vi "MCLB_AssertAllItems_Tests.vi"(11 "error in":errorcluster) -> (15 "error out":errorcluster)   [LabVIEW 2016, in "DronaTest.lvlib"]
uses:
  DronaTest.lvlib
  APIs/Stimulus/ControlValue/SetValueAuto.vi
  APIs/Assert/AssertControlValue/Controls/MC Listbox/AssertAllItems.vi
  <vilib>/addons/_JKI Toolkits/Caraya/classes/Assert/Assert Error.vi
  <vilib>/addons/_JKI Toolkits/Caraya/classes/Assert/Assert Equal Value_Variant.vi
  <vilib>/addons/_JKI Toolkits/Caraya/classes/Test/Test.lvclass
  Drona.lvlib
  <vilib>/SLL Toolkit/SLL Debug/SLL Debug.lvlib
  <vilib>/addons/_JKI Toolkits/Caraya/classes/Assert/Assert.lvclass
  APIs/Stimulus/ControlValue/ControlValue.lvlib
  APIs/Assert/AssertControlValue/Controls/MC Listbox/AssertMCListbox.lvlib
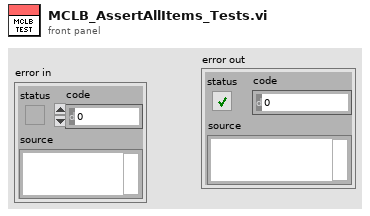
[diagram p1: front panel]
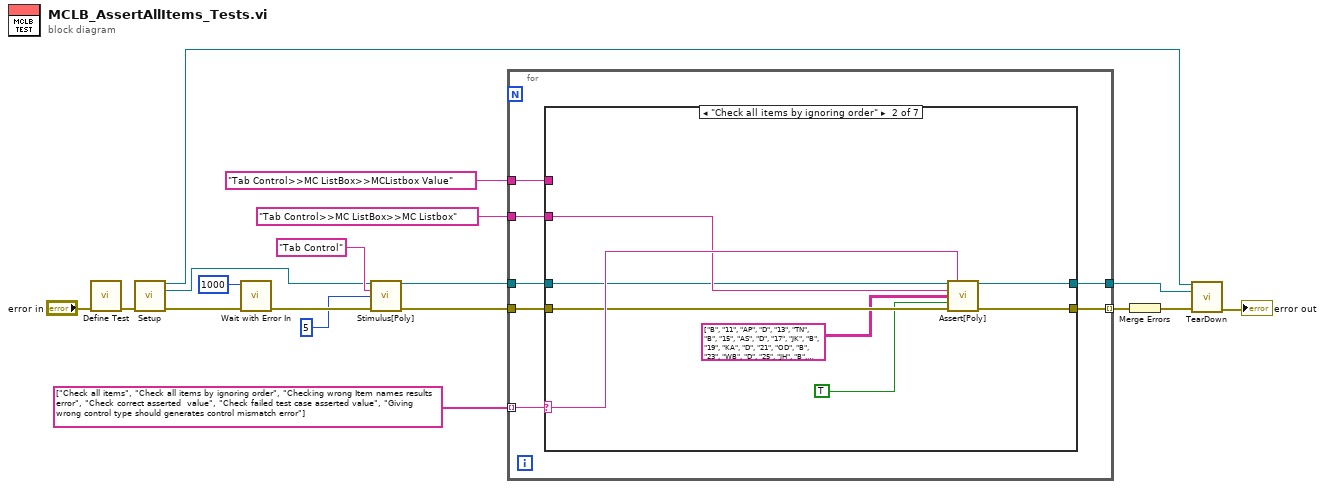
[diagram p0: block diagram]
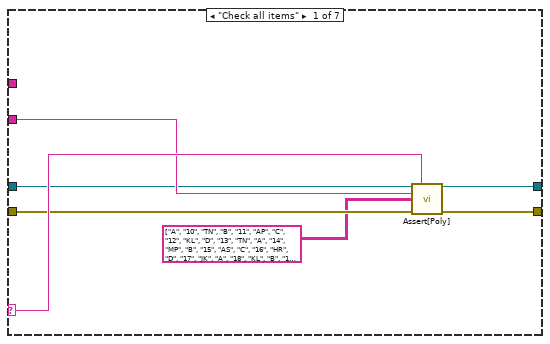
[diagram p2: hidden frame]
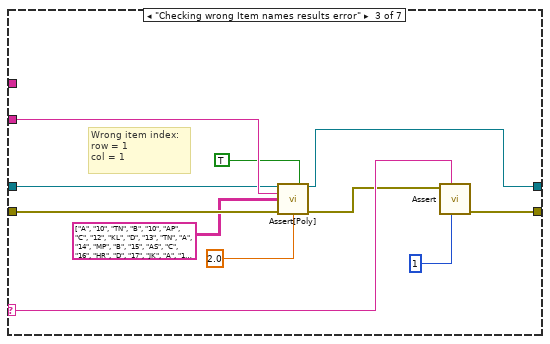
[diagram p3: hidden frame]
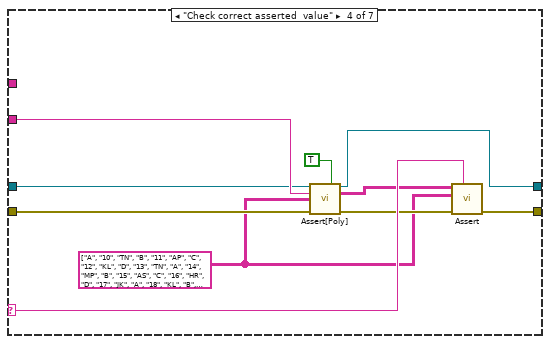
[diagram p4: hidden frame]
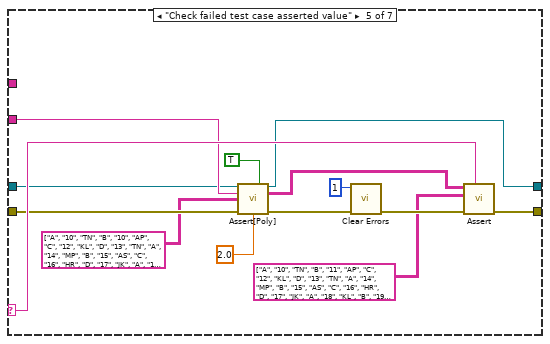
[diagram p5: hidden frame]
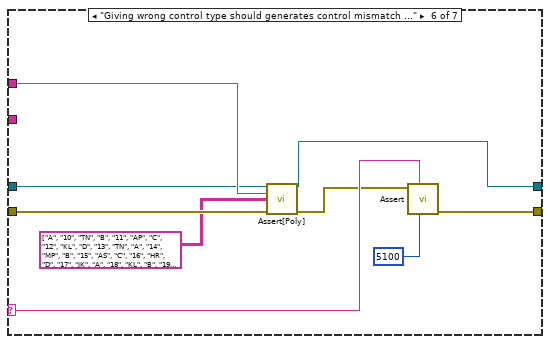
[diagram p6: hidden frame]
diagram:
  n1 = call <vilib>:"Define Test.vi"("error in (no error)"="error in") -> ("error out"=w7:errorcluster)  [unwired: 9 in, 1 out]
  n2 = call "Setup.vi"("error in (no error)"=w7) -> ("Application Ref"=w3:refnum<vi>, "VI out"=w5:refnum<vi>, "error out"=w6:errorcluster)  [unwired: 12 in]
  n3 = call <vilib>:"Wait with Error In.vi"("error in (no error)"=w6, "milliseconds to wait"=u32 1000) -> ("error out"=w16:errorcluster)  [unwired: 9 in]
  n4 = call-poly "Stimulus[Poly].vi"("VI Reference In"=w5, "Control Path"="Tab Control", "Value (Signaling)"=5, "error in"=w16) -> ("VI Reference Out"=w12:refnum<vi>, "error out"=w15:errorcluster)  [unwired: 10 in]
  n5 = for {
    tunnel: w12 -> [w24]
    tunnel: "Tab Control>>MC ListBox>>MC Listbox" ("Control Path") -> [w23]
    tunnel: "Tab Control>>MC ListBox>>MCListbox Value" ("Control Path") -> [w22]
    tunnel: string[] ["Check all items", "Check all items by ignoring order", "Checking wrong Item names results error", "Check correct asserted  value", "Check failed test case asserted value", "Giving wrong control type should generates control mismatch error"] -> [w20] mode=indexing
    tunnel: [w19] -> w2
    tunnel: w15 -> [w25]
    tunnel: [w21] -> w8 mode=indexing
    n6 = case shown="\"Check all items by ignoring order\"" w20 {
      selector: w20 -> [w30 w38 w50 w60 w74 w83 _]
      tunnel: w25 -> [w28 w36 w43 w56 w70 w78 w86]
      tunnel: w24 -> [w27 w35 w42 w55 w69 w77 w85]
      tunnel: w23 -> [w29 w37 w48 w59 w73 _ _]
      tunnel: w22 -> [_ _ _ _ _ w80 _]
      tunnel: [w32 w40 w51 w61 w75 w84 w86] -> w21
      tunnel: [w31 w39 w47 w58 w72 w79 w85] -> w19
      frame "Check all items" {
        n7 = call-poly "Assert[Poly].vi"("VI Reference In"=w27, "Test Label"=w30, "Control Path"=w29, "Item Names"=string[][] [["A", "10", "TN"], ["B", "11", "AP"], ["C", "12", "KL"], ["D", "13", "TN"], ["A", "14", "MP"], ["B", "15", "AS"], ["C", "16", "HR"], ["D", "17", "JK"], ["A", "18", "KL"], ["B", "19", "KA"], ["C", "20", "MH"], ["D", "21", "OD"], ["A", "22", "UP"], ["B", "23", "WB"], ["C", "24", "NL"], ["D", "25", "JH"], ["A", "26", "HP"], ["B", "27", "GJ"], ["C", "28", "GA"], ["D", "29", "BR"]], "Error In"=w28) -> ("VI Reference Out"=w31:refnum<vi>, "Error Out"=w32:errorcluster)  [unwired: 8 in, 1 out]
      }
      frame "Check all items by ignoring order" {
        n8 = call-poly "Assert[Poly].vi"("VI Reference In"=w35, "Test Label"=w38, "Control Path"=w37, "Item Names"=string[][] [["B", "11", "AP"], ["D", "13", "TN"], ["B", "15", "AS"], ["D", "17", "JK"], ["B", "19", "KA"], ["D", "21", "OD"], ["B", "23", "WB"], ["D", "25", "JH"], ["B", "27", "GJ"], ["D", "29", "BR"], ["A", "10", "TN"], ["C", "12", "KL"], ["A", "14", "MP"], ["C", "16", "HR"], ["A", "18", "KL"], ["C", "20", "MH"], ["A", "22", "UP"], ["C", "24", "NL"], ["A", "26", "HP"], ["C", "28", "GA"]], "Ignore Order? (F)"=TRUE, "Error In"=w36) -> ("VI Reference Out"=w39:refnum<vi>, "Error Out"=w40:errorcluster)  [unwired: 7 in, 1 out]
      }
      frame "Checking wrong Item names results error" {
        # "Wrong item index:\nrow = 1\ncol = 1"
        n9 = call-poly "Assert[Poly].vi"("VI Reference In"=w42, "Assert Only? (F)"=TRUE, "Control Path"=w48, "Item Names"=string[][] [["A", "10", "TN"], ["B", "10", "AP"], ["C", "12", "KL"], ["D", "13", "TN"], ["A", "14", "MP"], ["B", "15", "AS"], ["C", "16", "HR"], ["D", "17", "JK"], ["A", "18", "KL"], ["B", "19", "KA"], ["C", "20", "MH"], ["D", "21", "OD"], ["A", "22", "UP"], ["B", "23", "WB"], ["C", "24", "NL"], ["D", "25", "JH"], ["A", "26", "HP"], ["B", "27", "GJ"], ["C", "28", "GA"], ["D", "29", "BR"]], "Error In"=w43, "Timeout(5 sec)"=2.0) -> ("VI Reference Out"=w47:refnum<vi>, "Error Out"=w46:errorcluster)  [unwired: 7 in, 1 out]
        n10 = call-poly <vilib>:"Assert.vi"("error code (1)"=1, "Label"=w50, "Error?"=w46) -> ("error out"=w51:errorcluster)  [unwired: 7 in, 1 out]
      }
      frame "Check correct asserted  value" {
        w52 = string[][] [["A", "10", "TN"], ["B", "11", "AP"], ["C", "12", "KL"], ["D", "13", "TN"], ["A", "14", "MP"], ["B", "15", "AS"], ["C", "16", "HR"], ["D", "17", "JK"], ["A", "18", "KL"], ["B", "19", "KA"], ["C", "20", "MH"], ["D", "21", "OD"], ["A", "22", "UP"], ["B", "23", "WB"], ["C", "24", "NL"], ["D", "25", "JH"], ["A", "26", "HP"], ["B", "27", "GJ"], ["C", "28", "GA"], ["D", "29", "BR"]] ("Item Names")
        n11 = call-poly "Assert[Poly].vi"("VI Reference In"=w55, "Assert Only? (F)"=TRUE, "Control Path"=w59, "Item Names"=w52, "Error In"=w56) -> ("VI Reference Out"=w58:refnum<vi>, "Asserted Value"=w53:string[][], "Error Out"=w54:errorcluster)  [unwired: 8 in]
        n12 = call-poly <vilib>:"Assert.vi"("Label"=w60, "error in (no error)"=w54, "Y"=w52, "X"=w53) -> ("error out"=w61:errorcluster)  [unwired: 6 in, 1 out]
      }
      frame "Check failed test case asserted value" {
        n13 = call-poly "Assert[Poly].vi"("VI Reference In"=w69, "Assert Only? (F)"=TRUE, "Control Path"=w73, "Item Names"=string[][] [["A", "10", "TN"], ["B", "10", "AP"], ["C", "12", "KL"], ["D", "13", "TN"], ["A", "14", "MP"], ["B", "15", "AS"], ["C", "16", "HR"], ["D", "17", "JK"], ["A", "18", "KL"], ["B", "19", "KA"], ["C", "20", "MH"], ["D", "21", "OD"], ["A", "22", "UP"], ["B", "23", "WB"], ["C", "24", "NL"], ["D", "25", "JH"], ["A", "26", "HP"], ["B", "27", "GJ"], ["C", "28", "GA"], ["D", "29", "BR"]], "Error In"=w70, "Timeout(5 sec)"=2.0) -> ("VI Reference Out"=w72:refnum<vi>, "Asserted Value"=w67:string[][], "Error Out"=w68:errorcluster)  [unwired: 7 in]
        n14 = call <vilib>:"Clear Errors.vi"("error in (no error)"=w68, "specific error code to clear (0: all)"=1) -> ("error out"=w66:errorcluster)  [unwired: 4 in, 1 out]
        n15 = call-poly <vilib>:"Assert.vi"("Label"=w74, "error in (no error)"=w66, "Y"=string[][] [["A", "10", "TN"], ["B", "11", "AP"], ["C", "12", "KL"], ["D", "13", "TN"], ["A", "14", "MP"], ["B", "15", "AS"], ["C", "16", "HR"], ["D", "17", "JK"], ["A", "18", "KL"], ["B", "19", "KA"], ["C", "20", "MH"], ["D", "21", "OD"], ["A", "22", "UP"], ["B", "23", "WB"], ["C", "24", "NL"], ["D", "25", "JH"], ["A", "26", "HP"], ["B", "27", "GJ"], ["C", "28", "GA"], ["D", "29", "BR"]] ("Item Names"), "X"=w67) -> ("error out"=w75:errorcluster)  [unwired: 6 in, 1 out]
      }
      frame "Giving wrong control type should generates control mismatch error" {
        n16 = call-poly "Assert[Poly].vi"("VI Reference In"=w77, "Control Path"=w80, "Item Names"=string[][] [["A", "10", "TN"], ["B", "11", "AP"], ["C", "12", "KL"], ["D", "13", "TN"], ["A", "14", "MP"], ["B", "15", "AS"], ["C", "16", "HR"], ["D", "17", "JK"], ["A", "18", "KL"], ["B", "19", "KA"], ["C", "20", "MH"], ["D", "21", "OD"], ["A", "22", "UP"], ["B", "23", "WB"], ["C", "24", "NL"], ["D", "25", "JH"], ["A", "26", "HP"], ["B", "27", "GJ"], ["C", "28", "GA"], ["D", "29", "BR"]], "Error In"=w78) -> ("VI Reference Out"=w79:refnum<vi>, "Error Out"=w81:errorcluster)  [unwired: 9 in, 1 out]
        n17 = call-poly <vilib>:"Assert.vi"("error code (1)"=5100, "Label"=w83, "Error?"=w81) -> ("error out"=w84:errorcluster)  [unwired: 7 in, 1 out]
      }
      frame Default {
      }
    }
  }
  n18 = Merge Errors(w8) -> (w4:errorcluster)
  n19 = call "TearDown.vi"("Application Ref"=w3, "VI in"=w2, "error in (no error)"=w4) -> ("error out"=→"error out":errorcluster)  [unwired: 12 in]
